vi "Get AccessType.vi"(8 "Error In":errorcluster, 11 "reference in":refnum<class "OD Entry.lvclass">) -> (0 "Error Out":errorcluster, 2 "AccessType":T1=enum."const", 3 "reference out":refnum<class "OD Entry.lvclass">)   [LabVIEW 2024, in "EDS.lvlib" / "OD Entry.lvclass"]
uses:
  OD Entry.lvclass
  OD Entry.lvclass/OD Entry.ctl
  Access Type.ctl
  EDS.lvlib
panel:
  out "Defined?":bool
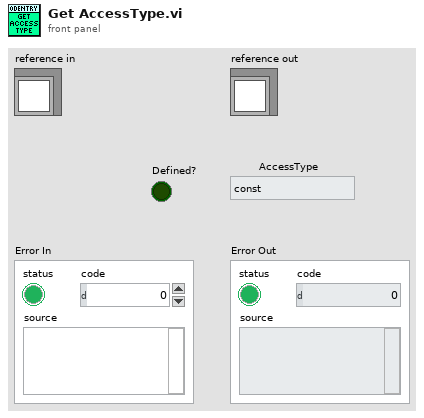
[diagram p1: front panel]
types:
  T1 = typedef "EDS.lvlib/Access Type.ctl" = enum16{"ro", "wo", "rw", "rwr", "rww", "const"}
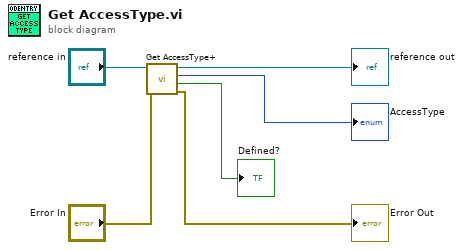
[diagram p0: block diagram]
diagram:
  n1 = call "Get AccessType+.vi"("Error In"="Error In", "reference in"="reference in") -> ("Error Out"=→"Error Out":errorcluster, "Defined?"=→"Defined?":bool, "AccessType"=→"AccessType":T1, "reference out"=→"reference out":refnum<class "OD Entry.lvclass">)  [unwired: 6 in]
